vi "CoinDetector2.vi"() -> ()   [LabVIEW 2020]
uses:
  <vilib>/Analysis/5stat.llb/RMS (DBL).vi
  <vilib>/Analysis/NI_AALPro.lvlib
panel:
  in  "Start":bool
  out "Now Freq":dbl
  out "Waveform Graph":dynamicdata(graph)
  out "Freq":dbl
  out "Freq":dbl
  out "Vout":dynamicdata(graph)
  out "RMS":dbl
  in  "stop":bool
  out "RMS":dbl
  out "Vin":dynamicdata(graph)
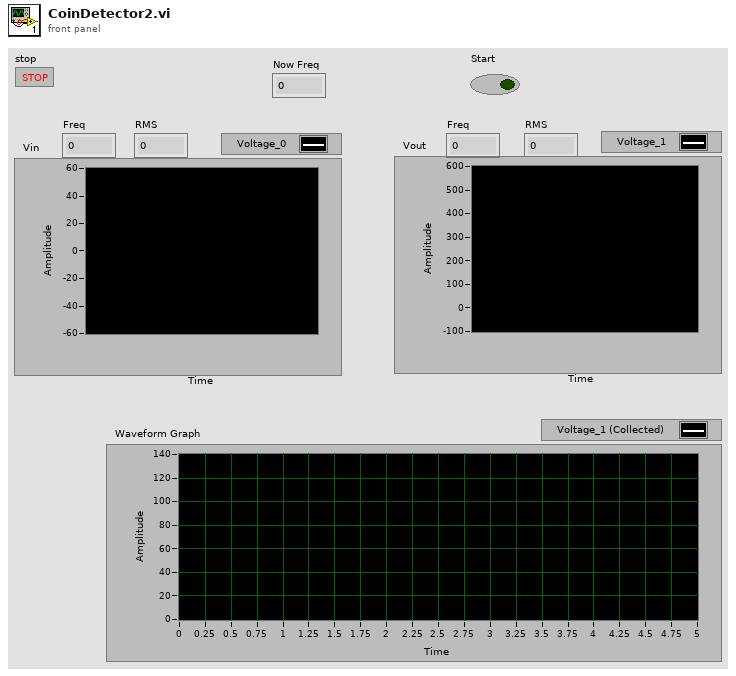
[diagram p1: front panel]
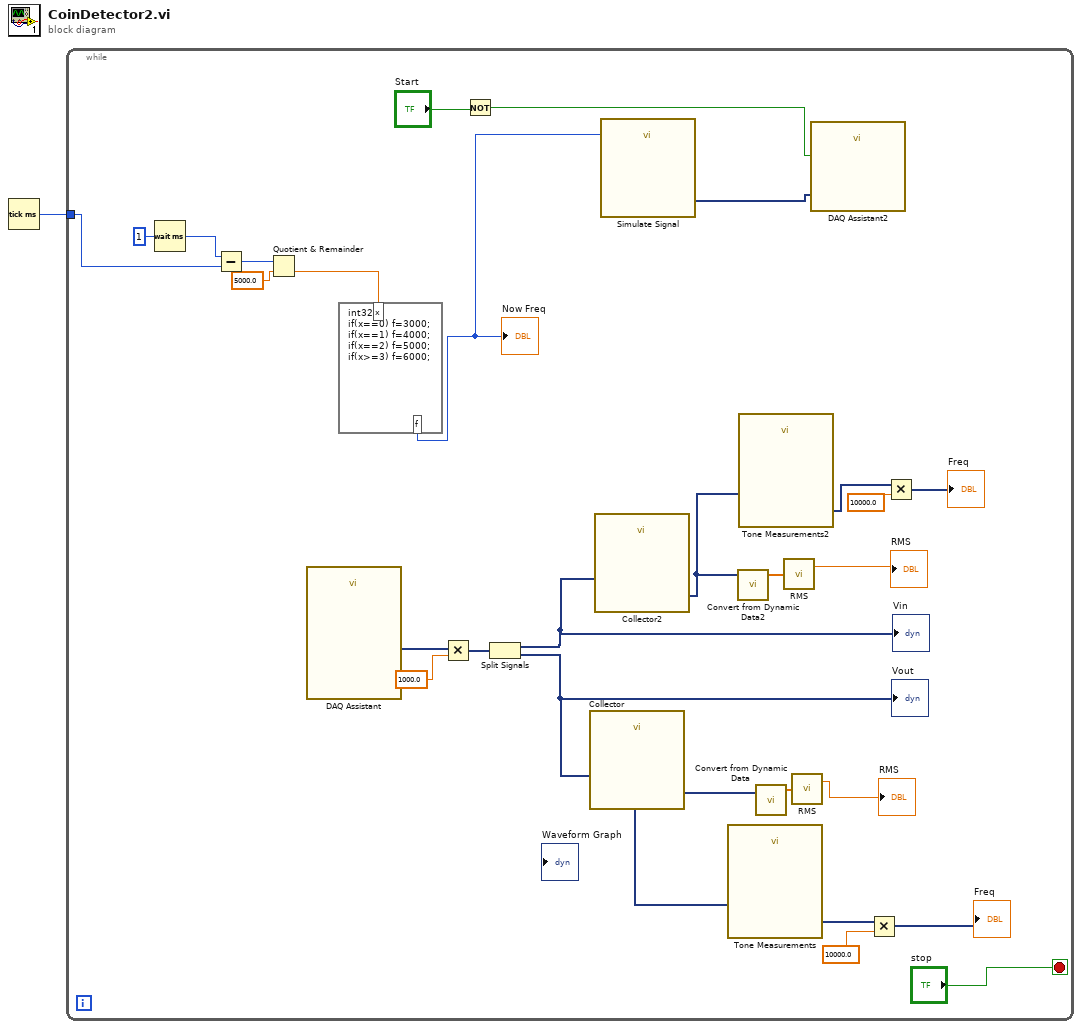
[diagram p0: block diagram]
diagram:
  n1 = Tick Count (ms)() -> (millisecond timer value=w1:u32)
  n2 = while {
    tunnel: w1 -> [w2]
    stop <- "stop" stop-if-true
    n3 = Wait (ms)(milliseconds to wait=u32 1) -> (millisecond timer value=w6:u32)
    n4 = Subtract(x=w6, y=w2) -> (x-y=w7:u32)
    n5 = Quotient & Remainder(x=w7, y=5000.0) -> (floor(x/y)=w8:dbl)  [unwired: 1 out]
    n6 = call "DAQ Assistant"() -> ("data"=w14:dynamicdata)  [unwired: 16 in, 3 out]
    n7 = formula code="int32 f;\nif(x==0) f=3000;\nif(x==1) f=4000;\nif(x==2) f=5000;\nif(x>=3) f=6000;"("x"=w8) -> ("f"=w9:i32)
    "Now Freq" <- w9
    n8 = Multiply(x=w14, y=1000.0) -> (x*y=w28:dynamicdata)
    n9 = Not(x="Start") -> (.not. x?=w11:bool)
    n10 = Split Signals(w28) -> (w21:dynamicdata, w25:dynamicdata)  [unwired: 2 in]
    "Vin" <- w21
    "Vout" <- w25
    n11 = call "Collector"("Signals"=w25) -> ("Collected Signals"=w13:dynamicdata)  [unwired: 9 in, 1 out]
    n12 = call "Collector2"("Signals"=w21) -> ("Collected Signals"=w18:dynamicdata)  [unwired: 9 in, 1 out]
    n13 = call "Simulate Signal"("Frequency"=w9) -> ("Sine"=w5:dynamicdata)  [unwired: 13 in, 1 out]
    n14 = call "Tone Measurements"("Signals"=w13) -> ("Frequency"=w22:dynamicdata)  [unwired: 9 in, 1 out]
    n15 = call "Convert from Dynamic Data2"("Dynamic Data Type"=w18) -> ("Array"=w20:dbl[])  [unwired: 3 in]
    n16 = call "Tone Measurements2"("Signals"=w18) -> ("Frequency"=w17:dynamicdata)  [unwired: 9 in, 1 out]
    n17 = call "Convert from Dynamic Data"("Dynamic Data Type"=w13) -> ("Array"=w27:dbl[])  [unwired: 3 in]
    n18 = call-poly <vilib>:"RMS.vi"("X"=w20) -> ("rms value"=→"RMS":dbl)  [unwired: 1 out]
    n19 = call-poly <vilib>:"RMS.vi"("X"=w27) -> ("rms value"=→"RMS":dbl)  [unwired: 1 out]
    n20 = call "DAQ Assistant2"("data"=w5, "stop (F)"=w11) -> ()  [unwired: 15 in, 3 out]
    n21 = Multiply(x=w22, y=10000.0) -> (x*y=→"Freq":dynamicdata)
    n22 = Multiply(x=w17, y=10000.0) -> (x*y=→"Freq":dynamicdata)
  }
